vi "工單號碼Cluster.vi"(11 "Cluster":T2) -> (3 "output cluster":T1)   [LabVIEW 2019]
panel:
  in  "Cluster 2":T1
  out "Total良率":string
  out "Operator":string
  out "品名":string
  out "產品料號":string
  out "Work No":string
  out "工單生產總數":string
  out "NG數量":string
  out "良品數量":string
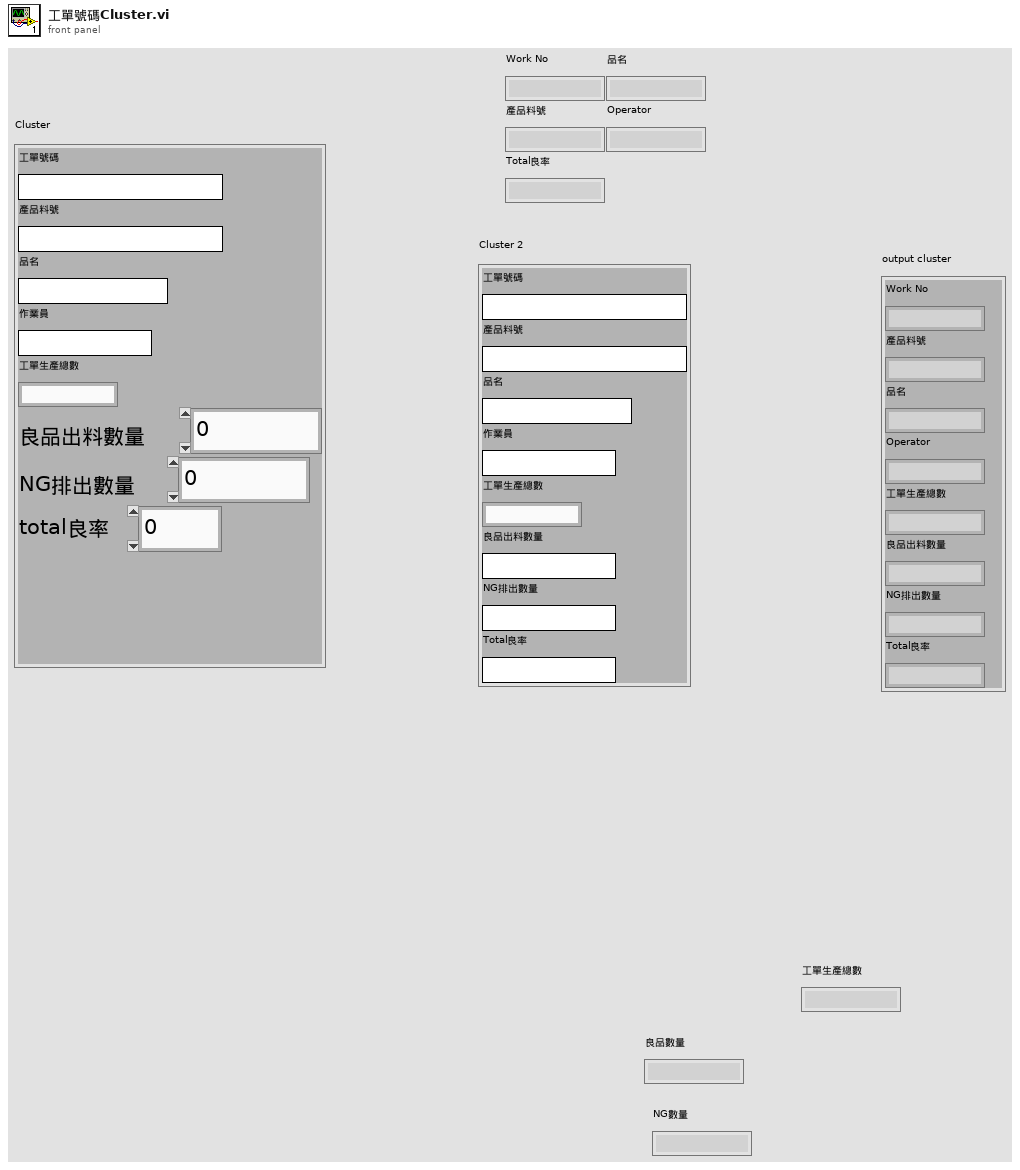
[diagram p1: front panel]
types:
  T1 = cluster{"Work No":string, "產品料號":string, "品名":string, "Operator":string, "工單生產總數":string, "良品出料數量":string, "NG排出數量":string, "Total良率":string}
  T2 = cluster{"Work No":string, "產品料號":string, "品名":string, "Operator":string, "工單生產總數":string, "良品出料數量":u16, "NG排出數量":u16, "total良率":u16}
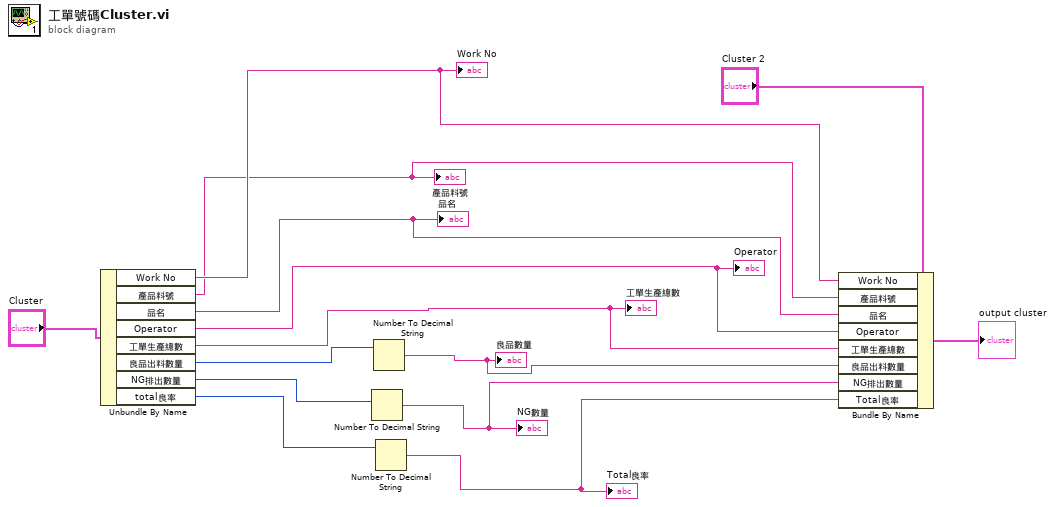
[diagram p0: block diagram]
diagram:
  n1 = Unbundle By Name("Cluster") -> ("Work No"=w13:string, "產品料號"=w11:string, "品名"=w10:string, "Operator"=w9:string, "工單生產總數"=w1:string, "良品出料數量"=w2:u16, "NG排出數量"=w3:u16, "total良率"=w4:u16)
  "工單生產總數" <- w1
  "Work No" <- w13
  "產品料號" <- w11
  "品名" <- w10
  "Operator" <- w9
  n2 = Number To Decimal String(number=w3) -> (decimal integer string=w7:string)  [unwired: 1 in]
  "NG數量" <- w7
  n3 = Number To Decimal String(number=w2) -> (decimal integer string=w8:string)  [unwired: 1 in]
  "良品數量" <- w8
  n4 = Number To Decimal String(number=w4) -> (decimal integer string=w6:string)  [unwired: 1 in]
  "Total良率" <- w6
  n5 = Bundle By Name(cluster="Cluster 2", "Work No"=w13, "產品料號"=w11, "品名"=w10, "Operator"=w9, "工單生產總數"=w1, "良品出料數量"=w8, "NG排出數量"=w7, "Total良率"=w6) -> (→"output cluster":T1)
